vi "Lorentzian.vi"(3 "output control":T1, 4 "data":T2, 5 "X":dbl[](array[numeric]), 6 "a":dbl[](array[numeric])) -> (0 "error out":errorcluster, 1 "f'(X,a)":dbl[][](array[numeric]), 2 "f(X,a)":dbl[](array[numeric]))   [LabVIEW 2010]
doc: "This template is the starting point for creating a model function to be passed to the Nonlinear Curve Fit.vi."
uses:
  <vilib>/gmath/NumericalOptimization/objective function data.ctl
  <vilib>/gmath/NumericalOptimization/LM_output select.ctl
  <vilib>/gmath/NI_Gmath.lvlib
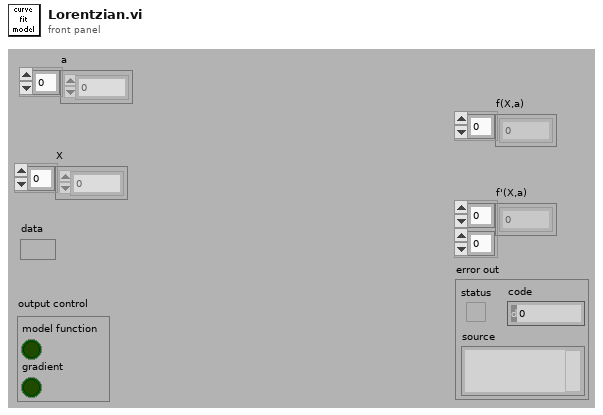
[diagram p1: front panel]
types:
  T1 = typedef "NI_Gmath.lvlib/LM_output select.ctl" = cluster{"model function":bool, "gradient":bool}
  T2 = typedef "NI_Gmath.lvlib/objective function data.ctl" = variant
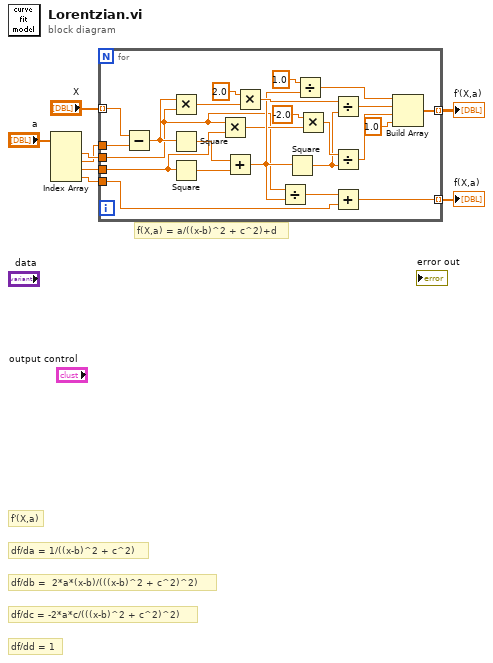
[diagram p0: block diagram]
diagram:
  # "f(X,a) = a/((x-b)^2 + c^2)+d"
  # "f'(X,a)"
  # "df/dd = 1"
  # "df/dc = -2*a*c/(((x-b)^2 + c^2)^2)"
  # "df/db =  2*a*(x-b)/(((x-b)^2 + c^2)^2)"
  # "df/da = 1/((x-b)^2 + c^2)"
  n1 = Index Array(array="a") -> (element #1=w4:dbl, element #2=w3:dbl, element #3=w2:dbl, element #4=w1:dbl)  [unwired: 4 in]
  n2 = for {
    tunnel: "X" -> [w29] mode=indexing
    tunnel: [w28] -> w7 mode=indexing
    tunnel: [w32] -> w6 mode=indexing
    tunnel: w4 -> [w13]
    tunnel: w3 -> [w30]
    tunnel: w2 -> [w12]
    tunnel: w1 -> [w27]
    n3 = Subtract(x=w29, y=w30) -> (x-y=w19:dbl)
    n4 = Multiply(x=w19, y=w13) -> (x*y=w20:dbl)
    n5 = Square(x=w19) -> (x^2=w26:dbl)
    n6 = Square(x=w12) -> (x^2=w25:dbl)
    n7 = Multiply(x=w13, y=w12) -> (x*y=w14:dbl)
    n8 = Add(x=w26, y=w25) -> (x+y=w17:dbl)
    n9 = Multiply(x=2.0, y=w20) -> (x*y=w18:dbl)
    n10 = Divide(x=w13, y=w17) -> (x/y=w24:dbl)
    n11 = Square(x=w17) -> (x^2=w10:dbl)
    n12 = Divide(x=1.0, y=w17) -> (x/y=w22:dbl)
    n13 = Multiply(x=-2.0, y=w14) -> (x*y=w11:dbl)
    n14 = Divide(x=w18, y=w10) -> (x/y=w16:dbl)
    n15 = Divide(x=w11, y=w10) -> (x/y=w9:dbl)
    n16 = Add(x=w24, y=w27) -> (x+y=w28:dbl)
    n17 = Build Array(w22, w16, w9, 1.0) -> (w32:dbl[])
  }
  "f(X,a)" <- w7
  "f'(X,a)" <- w6
